vi "Calibration Parameters to text array.vi"(10 "Calibration Parameters":T1[](array[typedef]), 11 "Image No":string[](array[string])) -> (3 "Calibration Parameters":string[][](array[string]))   [LabVIEW 2020]
uses:
  TypeDefs/Current Calibration Parameters.ctl
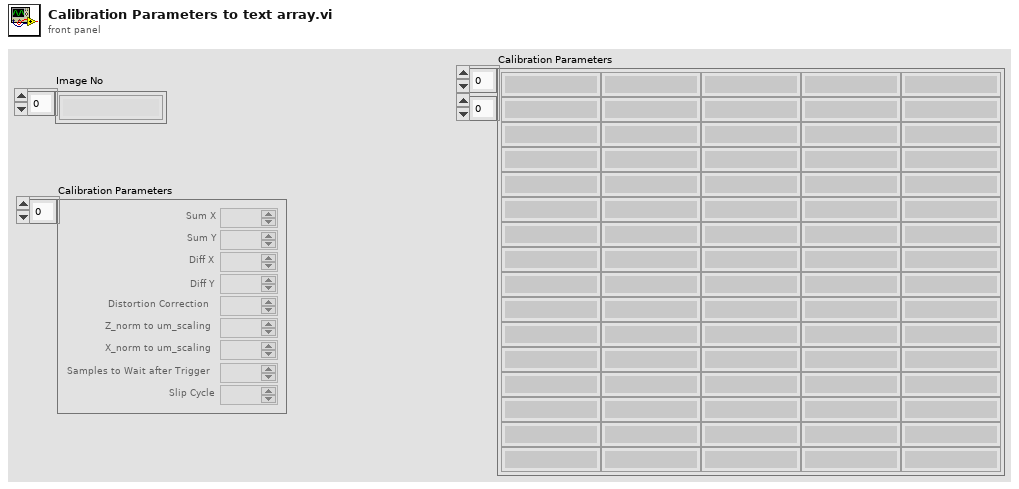
[diagram p1: front panel]
types:
  T1 = typedef "Current Calibration Parameters.ctl" = cluster{"Sum X":dbl, "Sum Y":dbl, "Diff X":dbl, "Diff Y":dbl, "Distortion Correction":dbl, "Z_norm to um_scaling":dbl, "X_norm to um_scaling":dbl, "Samples to Wait after Trigger":dbl, "Slip Cycle":dbl}
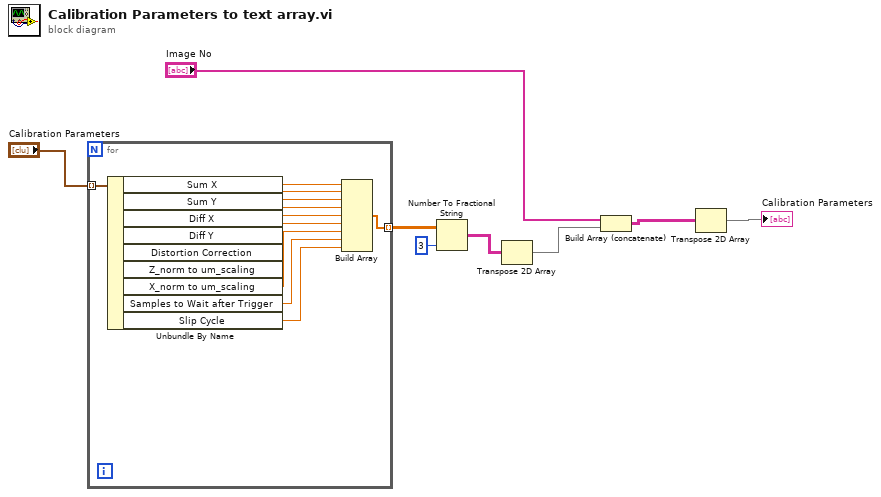
[diagram p0: block diagram]
diagram:
  n1 = for {
    tunnel: "Calibration Parameters" -> [w19] mode=indexing
    tunnel: [w9] -> w8 mode=indexing
    n2 = Unbundle By Name(w19) -> ("Sum X"=w18:dbl, "Sum Y"=w17:dbl, "Diff X"=w16:dbl, "Diff Y"=w15:dbl, "Distortion Correction"=w14:dbl, "Z_norm to um_scaling"=w13:dbl, "X_norm to um_scaling"=w12:dbl, "Samples to Wait after Trigger"=w11:dbl, "Slip Cycle"=w10:dbl)
    n3 = Build Array(w18, w17, w16, w15, w14, w13, w12, w11, w10) -> (w9:dbl[])
  }
  n4 = Number To Fractional String(number=w8, precision (6)=i16 3) -> (F-format string=w5:string[][])  [unwired: 2 in]
  n5 = Transpose 2D Array(2D array=w5) -> (transposed array=w4:string[][])
  n6 = Build Array (concatenate)("Image No", w4) -> (w3:string[][])
  n7 = Transpose 2D Array(2D array=w3) -> (transposed array=→"Calibration Parameters":string[][])
